vi "Hikvision 4004Hc EyeTraker.vi"() -> ()   [LabVIEW 2011]
uses:
  <vilib>/picture/picture.llb/imagedata.ctl
  <vilib>/Platform/TimedLoop/XDataNode/timing_clust.ctl
  <vilib>/Platform/TimedLoop/XDataNode/nitl_modes.ctl
  <vilib>/Platform/TimedLoop/XDataNode/wakeup.ctl
  <vilib>/Utility/file.llb/Read From Spreadsheet File (DBL).vi
  <vilib>/Utility/config.llb/Read Key (I32).vi
  <vilib>/Utility/config.llb/Read Key (U32).vi
  <vilib>/Utility/file.llb/Write To Spreadsheet File (DBL).vi
  <vilib>/Utility/config.llb/Write Key (I32).vi
  <vilib>/Utility/config.llb/Write Key (U32).vi
  <vilib>/Platform/TimedLoop/XDataNode/XDataNode.xnode
  <vilib>/Platform/TimedLoop/XDataNode/XDNodeRunTimeDep.lvlib
  <vilib>/Utility/config.llb/NI_LVConfig.lvlib
  <vilib>/vision/NI_Vision_Development_Module.lvlib
panel:
  out "XY图":cluster{dbl[], dbl[]}(graph)
  out "Histogram Graph":T1(graph) caption="直方图"
  in  "AviFileName":string="test9dots.avi"
  in  "method":enum16{"pupil", "CR", "pupil-CR"}(ring)=enum."pupil-CR"
  in  "bin":i32=10
  out "Frame Number":u32
  out "rectangle1":T2
  out "rectangle2":T2
  out "Image 2":T3(plugin-control)
  out "Image":T3(plugin-control)
  in  "VideoPara":cluster{"Brightness":i32, "Contrast":i32}={"Brightness"=128, "Contrast"=64} {"Contrast" min=0 max=127 scale=0.0..127.0; "Brightness" min=0 max=255 scale=0.0..255.0}
  out "valid fit 2":cluster{"CR Fit":bool, "pupil Fit":bool}
  out "valid fit":cluster{"CR Fit":bool, "pupil Fit":bool}
  in  "gaze Threshold1":dbl=2.0
  out "RAW循环持续时间":u64
  in  "blank of eye":T4={"NO. of Eyes"=0, "单选按钮"=enum."单选选项1", "eye1"=16711680, "eye2"=6618880} {"NO. of Eyes" items=["OneEye", "TwoEyes"]}
  out "数据处理循环持续时间 2":u64
  in  "CR Threshold 2":u8=240
  in  "Pupil Threshold 2":u8=75
  out "eye2":picture caption="新图片"
  in  "gaze Threshold 2":dbl=2.0
  out "gazing 2":bool
  in  "ImgResourse":u16(ring) items=["realeye", "avi"]
  out "gazing1":bool
  in  "Pupil Threshold1":u8=75
  in  "CR Threshold1":u8=240
  out "数据处理循环持续时间1":u64
  out "eye1":picture caption="新图片"
  out "new picture":picture caption="新图片"
  out "ROI循环持续时间":u64
  in  "停止":bool
  out "返回类型":i32
  out "ChannelOpen":u32 format="%x"
  out "GetTotalChannels":i32
  out "InitDSPs":i32
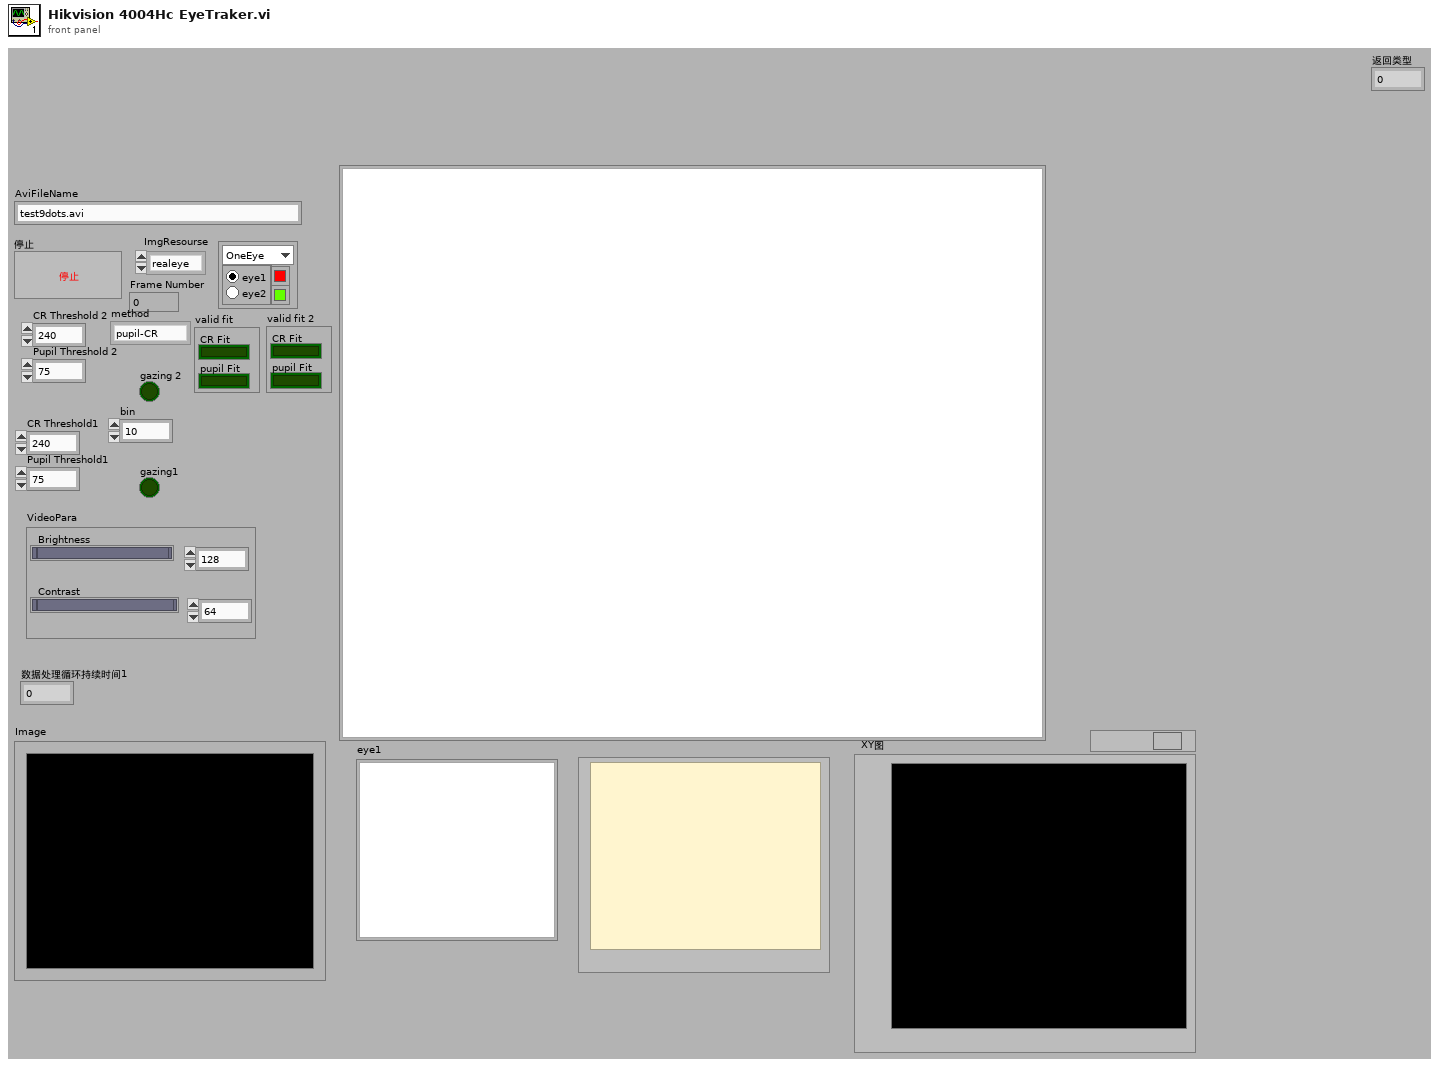
[diagram p1: front panel]
types:
  T1 = cluster{"X Values":dbl[], "Histogram: h(x)":i32[]}
  T2 = cluster{"value":i32, "value":i32, "value":i32, "value":i32}
  T3 = typedef "IMAQ Image.ctl" = refnum<image>
  T4 = cluster{"NO. of Eyes":u16, "单选按钮":enum32{"单选选项1", "单选选项2"}, "eye1":u32, "eye2":u32}
  T5 = typedef "XDNodeRunTimeDep.lvlib/timing_clust.ctl" = cluster{"Expected End [f-1]":u64, "Actual End [f-1]":u64, "Finished Late? [f-1]":bool, "Expected End [i-1]":u64, "Actual End [i-1]":u64, "Finished Late? [i-1]":bool, "Expected Start [i]":u64, "Actual Start [i]":u64, "Expected Start [f]":u64, "Actual Start [f]":u64, "Source Name":string, "Structure Name":string, "Period":i64, "Deadline":i64, "Offset":i64, "Start":i64, "Priority":i32, "Timeout":i32, "Mode":T6, "Wakeup Reason":T7, "Error":errorcluster, "Source Type":string, "Secondary Source Type":string, "Global End Time":u64, "Global Start Time":u64, "Frame Duration":u64, "Iteration Duration":u64, "Assigned CPU":i32, "I/O Scan Engine Mode":u32}
  T6 = typedef "XDNodeRunTimeDep.lvlib/nitl_modes.ctl" = enum32{"No Change", "Process missed periods, maintain original phase", "Discard missed periods, maintain original phase", "Process missed periods, ignore original phase", "Discard missed periods, ignore original phase"}
  T7 = typedef "XDNodeRunTimeDep.lvlib/wakeup.ctl" = enum32{"Normal", "Aborted", "Asynchronous wakeup", "Timing source error", "Timed loop error", "Timeout"}
  T8 = cluster{"pupil-CR array output":cluster{dbl[], dbl[]}, "CR array output":cluster{dbl[], dbl[]}, "pupil array output 3":cluster{dbl[], dbl[]}}
  T9 = typedef "NI_LVConfig.lvlib/Config Data RefNum.ctl" = refnum<k1>
  T10 = cluster{"ScreenWidth":i32, "ScreenHeight":i32, "distance":i32, "CameraDistance":i32, "AngleX":i32, "AngleY":i32}
  T11 = cluster{"CR":dbl[][], "pupil":dbl[][], "pupil-CR":dbl[][]}
  T12 = cluster{"CR":cluster{"平移参数":cluster{dbl, dbl}, "旋转参数":dbl, "y轴调整":dbl, "x曲面调整":dbl, "y曲面调整":dbl}, "pupil":cluster{"平移参数":cluster{dbl, dbl}, "旋转参数":dbl, "y轴调整":dbl, "x曲面调整":dbl, "y曲面调整":dbl}, "pupil-CR":cluster{"平移参数":cluster{dbl, dbl}, "旋转参数":dbl, "y轴调整":dbl, "x曲面调整":dbl, "y曲面调整":dbl}}
  T13 = typedef "Image Type" = u32
  T14 = typedef "imagedata.ctl" = cluster{"image type":i32, "image depth":i32, "image":u8[], "mask":u8[], "colors":u32[], "Rectangle":cluster{"left":i16, "top":i16, "right":i16, "bottom":i16}}
  T15 = cluster{"image subset":T14, "image subset":T14, bool}
  T16 = cluster{"CR Valid Fit":bool, "pupil Valid Fit":bool}
  T17 = cluster{"Minor Axis":cluster{"Point 1":cluster{"X":sgl, "Y":sgl}, "Point 2":cluster{"X":sgl, "Y":sgl}}, "Major Axis":cluster{"Point 1":cluster{"X":sgl, "Y":sgl}, "Point 2":cluster{"X":sgl, "Y":sgl}}, "输出簇":cluster{"point":cluster{"X":i32, "Y":i32}[], "Center":cluster{"X":sgl, "Y":sgl}}}
  T18 = cluster{"Point 1":cluster{"X":sgl, "Y":sgl}, "Point 2":cluster{"X":sgl, "Y":sgl}}
  T19 = typedef "AviRefnum.ctl" = refnum<k1>
  T20 = typedef "eventvkey.ctl" = enum16{"ASCII", "Enter", "Return", "Shift", "Ctrl", "Alt", "Cmd", "Opt", "Caps", "NumLock", "Clear", "Break", "Up", "Down", "Left", "Right", "Insert", "Delete", "Home", "End", "PageUp", "PageDown", "Escape", "Help", "Pause", "ScrollLock", "F1", "F2", "F3", "F4", "F5", "F6", "F7", "F8", "F9", "F10", "F11", "F12", "F13", "F14", "F15", "F16", "F17", "F18", "F19", "F20", "F21", "F22", "F23", "F24", "Play", "VolumeUp", "VolumeDown", "Mute", "Two Byte Char"}
  T21 = typedef "LVMouseTypeDef.ctl" = cluster{"Mouse Position":cluster{"X":i32, "Y":i32}, "Mouse Modifiers":cluster{"Button Down":bool, "Shift Mod":bool, "Menu Mod":bool, "Option Mod":bool}}
  T22 = cluster{"image subset":T14, "image subset":T14, "停止":bool}
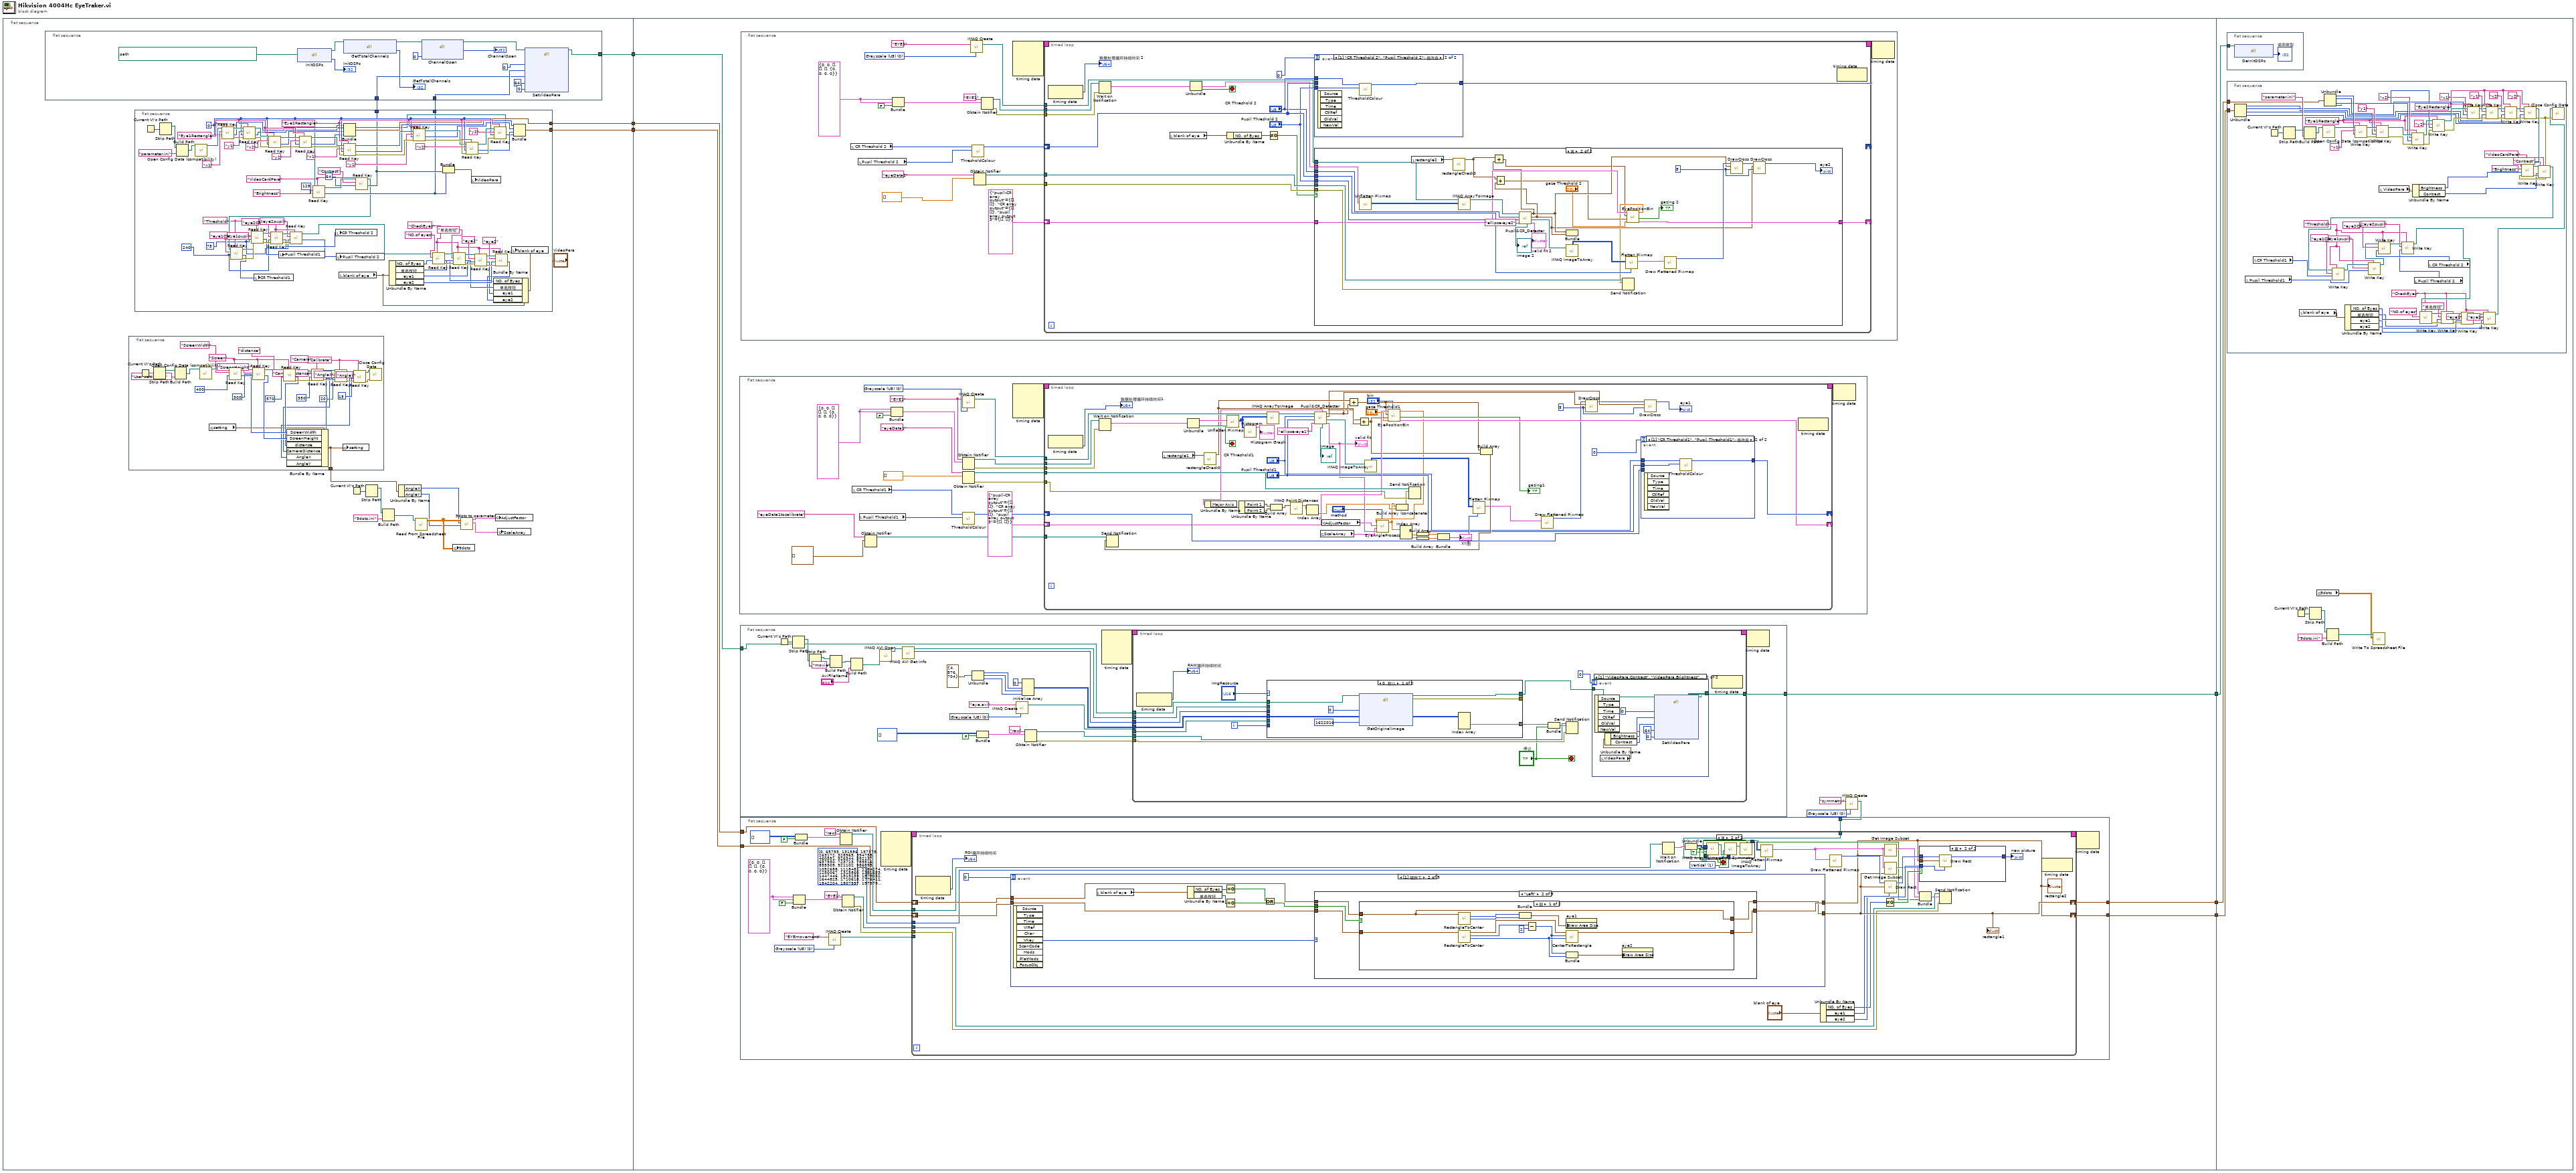
[diagram p0: block diagram]
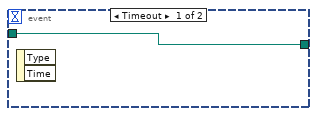
[diagram p2: hidden frame]
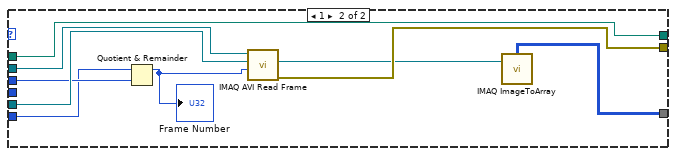
[diagram p3: hidden frame]
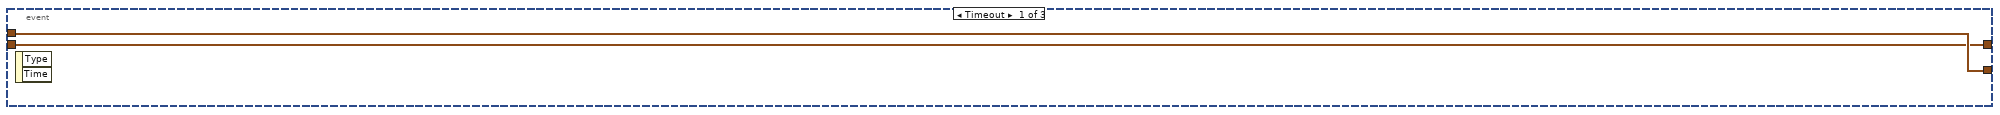
[diagram p6: hidden frame]
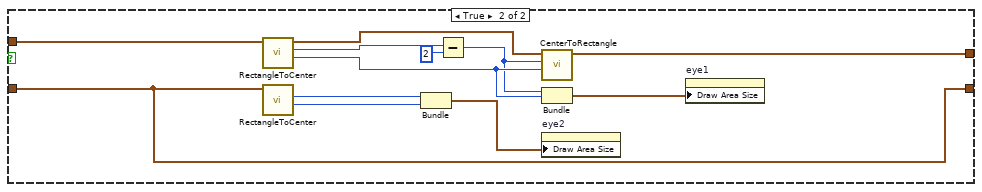
[diagram p8: hidden frame]
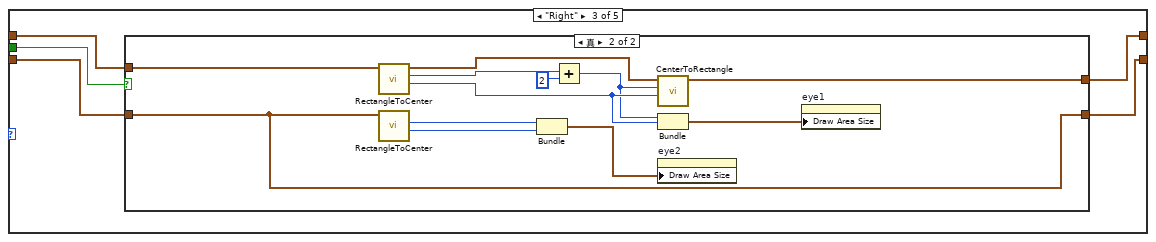
[diagram p9: hidden frame]
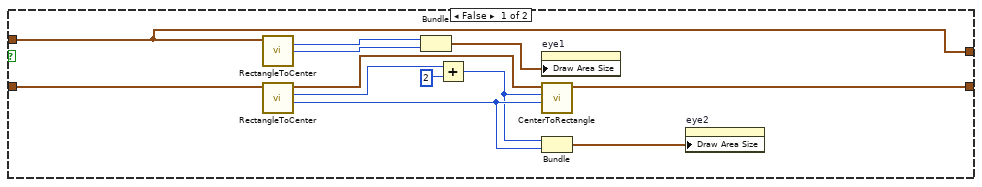
[diagram p10: hidden frame]
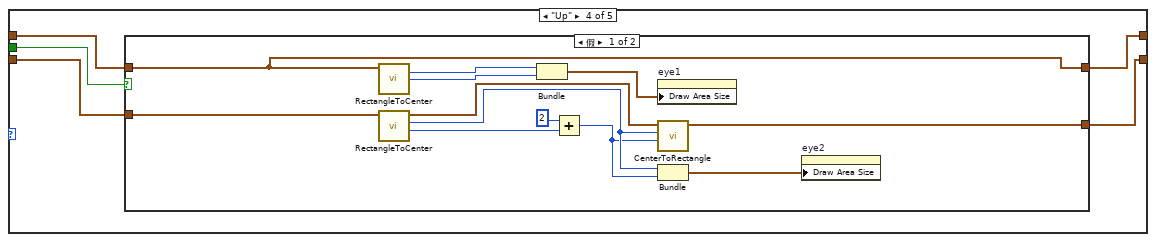
[diagram p11: hidden frame]
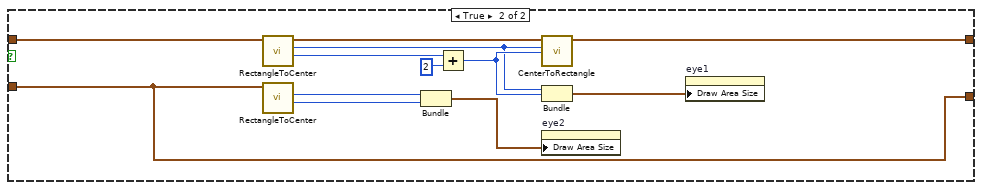
[diagram p12: hidden frame]
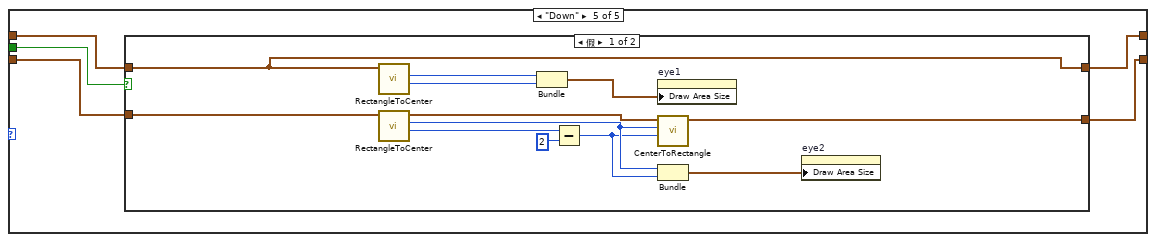
[diagram p13: hidden frame]
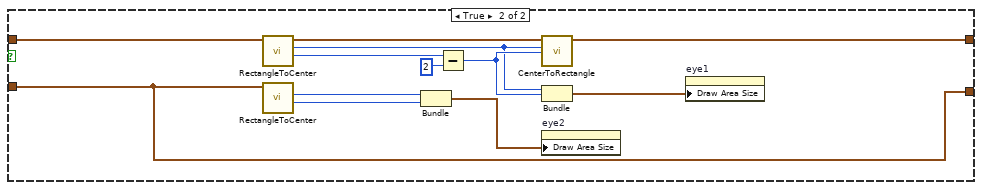
[diagram p14: hidden frame]
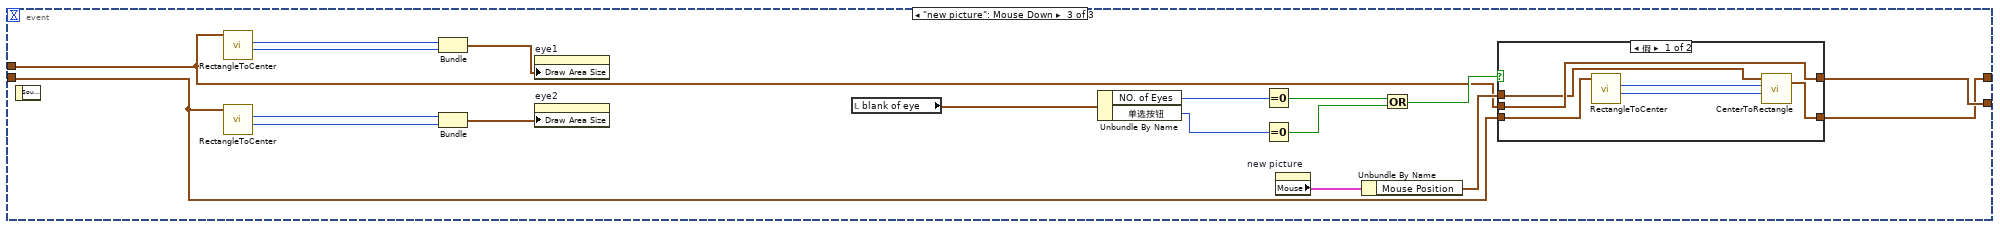
[diagram p15: hidden frame]
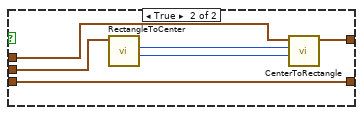
[diagram p16: hidden frame]
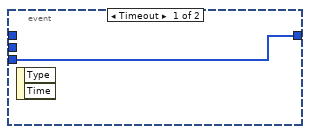
[diagram p17: hidden frame]
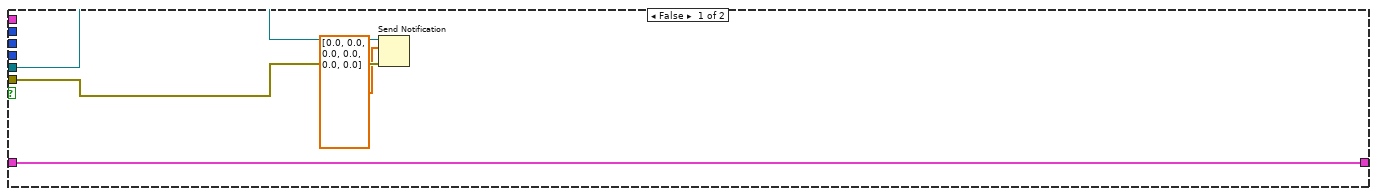
[diagram p18: hidden frame]
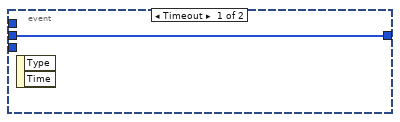
[diagram p19: hidden frame]
diagram:
  n1 = flat-sequence {
    tunnel: [w21] -> w6
    tunnel: [w20] -> w3
    tunnel: [w19] -> w2
    tunnel: w6 -> [w168]
    tunnel: [w172] -> w5
    tunnel: [w171] -> w4
    tunnel: w3 -> [w170]
    tunnel: w2 -> [w169]
    tunnel: [w167] -> w1
    tunnel: w5 -> [w654]
    tunnel: w4 -> [w653]
    tunnel: w1 -> [w652]
    frame #0 {
      n2 = flat-sequence {
        tunnel: [w66] -> w21
        tunnel: w18 -> [w60]
        tunnel: w17 -> [w61]
        frame #0 {
          n3 = dll-call lib="PTH1]abs CDocuments and Settingspan桌面workeye tracker\nHikvision Dll\nDs40xxSDK.dll" fn="InitDSPs"(path in=path "C:/Program Files/Hikvision/DS-4000系列板卡SDK and Demo Version 5.1/SDK/card sdk/Ds40xxSDK.dll" ("dll路径输入")) -> (path out=w68:path, "返回类型"=→"InitDSPs":i32)  [unwired: 2 in, 1 out]
          n4 = dll-call lib="PTH1]abs CDocuments and Settingspan桌面workeye tracker\nHikvision Dll\nDs40xxSDK.dll" fn="GetTotalChannels"(path in=w68) -> (path out=w70:path, "返回类型"=→"GetTotalChannels":i32)  [unwired: 2 in, 1 out]
          n5 = dll-call lib="PTH1]abs CDocuments and Settingspan桌面workeye tracker\nHikvision Dll\nDs40xxSDK.dll" fn="ChannelOpen"(path in=w70, "ChannelNum"=0) -> (path out=w65:path, "返回类型"=→"ChannelOpen":u32)  [unwired: 3 in, 1 out]
          n6 = dll-call lib="PTH1babs C\nProgram Files\tHikvision+DS-4000系列板卡SDK and Demo Version 5.1Bin\nDs40xxSDK.dll" fn="SetVideoPara"(path in=w65, "hChannelHandle"=u32 0, "Brightness"=w61, "Contrast"=w60, "Saturation"=64, "Hue"=0) -> (path out=w66:path)  [unwired: 7 in, 2 out]
        }
      }
      n7 = flat-sequence {
        tunnel: [w23] -> w9
        frame #0 {
          w30 = "Calibrate" ("section")
          w49 = "Screen" ("section")
          n8 = Current VI's Path() -> (path=w58:path)
          n9 = Strip Path(path=w58) -> (stripped path=w59:path)  [unwired: 1 out]
          n10 = Build Path(base path=w59, name or relative path="User Setting.ini" ("名称或相对路径")) -> (appended path=w56:path)
          n11 = call <vilib>:"Open Config Data (compatibility).vi"("configuration file path"=w56) -> ("refnum"=w55:T9)  [unwired: 8 in, 2 out]
          n12 = global read "全局 1.vi" "setting"() -> (w22:T10)
          n13 = call-poly <vilib>:"Read Key.vi"("section"=w49, "default value"=400 ("Pupil Threshold1"), "key"="ScreenWidth", "refnum"=w55) -> ("value"=w40:i32, "refnum out"=w53:T9)  [unwired: 1 in, 5 out]
          n14 = call-poly <vilib>:"Read Key.vi"("section"=w49, "default value"=300 ("Pupil Threshold1"), "key"="ScreenHeight", "refnum"=w53) -> ("value"=w39:i32, "refnum out"=w52:T9)  [unwired: 1 in, 5 out]
          n15 = call-poly <vilib>:"Read Key.vi"("section"=w49, "default value"=570 ("Pupil Threshold1"), "key"="distance", "refnum"=w52) -> ("error out"=w47:errorcluster, "value"=w38:i32, "refnum out"=w48:T9)  [unwired: 1 in, 4 out]
          n16 = call-poly <vilib>:"Read Key.vi"("section"="Camera", "error in (no error)"=w47, "default value"=350 ("Pupil Threshold1"), "key"="CameraDistance", "refnum"=w48) -> ("error out"=w37:errorcluster, "value"=w36:i32, "refnum out"=w35:T9)  [unwired: 4 out]
          n17 = call-poly <vilib>:"Read Key.vi"("section"=w30, "error in (no error)"=w37, "default value"=20 ("Pupil Threshold1"), "key"="AngleX", "refnum"=w35) -> ("error out"=w33:errorcluster, "value"=w25:i32, "refnum out"=w34:T9)  [unwired: 4 out]
          n18 = call-poly <vilib>:"Read Key.vi"("section"=w30, "error in (no error)"=w33, "default value"=15 ("Pupil Threshold1"), "key"="AngleY", "refnum"=w34) -> ("error out"=w31:errorcluster, "value"=w24:i32, "refnum out"=w32:T9)  [unwired: 4 out]
          n19 = Bundle By Name(cluster=w22, "ScreenWidth"=w40, "ScreenHeight"=w39, "distance"=w38, "CameraDistance"=w36, "AngleX"=w25, "AngleY"=w24) -> (w23:T10)
          n20 = global write "全局 1.vi" "setting"(w23) -> ()
          n21 = call <vilib>:"Close Config Data.vi"("error in (no error)"=w31, "refnum"=w32) -> ()  [unwired: 1 in, 9 out]
        }
      }
      n22 = flat-sequence {
        tunnel: [w125] -> w20
        tunnel: [w124] -> w19
        tunnel: [w116] -> w18
        tunnel: [w115] -> w17
        frame #0 {
          w74 = "CheckEyes" ("section")
          w98 = 75
          w100 = 240
          w106 = "Threshold" ("section")
          w121 = "VideoCardPara" ("section")
          w134 = 0
          w153 = "Eye2Rectangle" ("section")
          w148 = "Eye1Rectangle" ("section")
          n23 = Current VI's Path() -> (path=w135:path)
          n24 = Strip Path(path=w135) -> (stripped path=w136:path)  [unwired: 1 out]
          n25 = Build Path(base path=w136, name or relative path="parameter.ini" ("名称或相对路径")) -> (appended path=w138:path)
          n26 = call <vilib>:"Open Config Data (compatibility).vi"("configuration file path"=w138) -> ("refnum"=w139:T9)  [unwired: 8 in, 2 out]
          n27 = call-poly <vilib>:"Read Key.vi"("section"=w148, "default value"=w134, "key"="x1", "refnum"=w139) -> ("error out"=w141:errorcluster, "value"=w133:i32, "refnum out"=w142:T9)  [unwired: 1 in, 4 out]
          n28 = call-poly <vilib>:"Read Key.vi"("section"=w148, "error in (no error)"=w141, "default value"=w134, "key"="y1", "refnum"=w142) -> ("error out"=w144:errorcluster, "value"=w132:i32, "refnum out"=w145:T9)  [unwired: 4 out]
          n29 = call-poly <vilib>:"Read Key.vi"("section"=w148, "error in (no error)"=w144, "default value"=w134, "key"="x2", "refnum"=w145) -> ("error out"=w146:errorcluster, "value"=w131:i32, "refnum out"=w147:T9)  [unwired: 4 out]
          n30 = call-poly <vilib>:"Read Key.vi"("section"=w148, "error in (no error)"=w146, "default value"=w134, "key"="y2", "refnum"=w147) -> ("error out"=w163:errorcluster, "value"=w130:i32, "refnum out"=w162:T9)  [unwired: 4 out]
          n31 = local read "blank of eye"() -> (w81:T4)
          n32 = Bundle("value"=w133, "value"=w132, "value"=w131, "value"=w130) -> (w125:T2)  [unwired: 1 out]
          n33 = call-poly <vilib>:"Read Key.vi"("section"=w153, "error in (no error)"=w163, "default value"=w134, "key"="x1", "refnum"=w162) -> ("error out"=w160:errorcluster, "value"=w129:i32, "refnum out"=w159:T9)  [unwired: 4 out]
          n34 = Unbundle By Name(w81) -> ("NO. of Eyes"=w85:u16, "单选按钮"=w84:enum32{"单选选项1", "单选选项2"}, "eye1"=w83:u32, "eye2"=w82:u32)
          n35 = call-poly <vilib>:"Read Key.vi"("section"=w153, "error in (no error)"=w160, "default value"=w134, "key"="y1", "refnum"=w159) -> ("error out"=w157:errorcluster, "value"=w128:i32, "refnum out"=w156:T9)  [unwired: 4 out]
          n36 = call-poly <vilib>:"Read Key.vi"("section"=w153, "error in (no error)"=w157, "default value"=w134, "key"="x2", "refnum"=w156) -> ("error out"=w155:errorcluster, "value"=w127:i32, "refnum out"=w154:T9)  [unwired: 4 out]
          n37 = call-poly <vilib>:"Read Key.vi"("section"=w153, "error in (no error)"=w155, "default value"=w134, "key"="y2", "refnum"=w154) -> ("value"=w126:i32, "refnum out"=w123:T9)  [unwired: 5 out]
          n38 = call-poly <vilib>:"Read Key.vi"("section"=w121, "default value"=128, "key"="Brightness", "refnum"=w123) -> ("value"=w115:i32, "refnum out"=w120:T9)  [unwired: 1 in, 5 out]
          n39 = call-poly <vilib>:"Read Key.vi"("section"=w121, "default value"=64, "key"="Contrast", "refnum"=w120) -> ("value"=w116:i32, "refnum out"=w107:T9)  [unwired: 1 in, 5 out]
          n40 = call-poly <vilib>:"Read Key.vi"("section"=w106, "default value"=w100, "key"="eye1CR", "refnum"=w107) -> ("error out"=w113:errorcluster, "value"=w103:i32, "refnum out"=w112:T9)  [unwired: 1 in, 4 out]
          n41 = call-poly <vilib>:"Read Key.vi"("section"=w106, "error in (no error)"=w113, "default value"=w98, "key"="eye1pupil", "refnum"=w112) -> ("error out"=w111:errorcluster, "value"=w102:i32, "refnum out"=w110:T9)  [unwired: 4 out]
          n42 = local write "CR Threshold1"(w103) -> ()
          n43 = call-poly <vilib>:"Read Key.vi"("section"=w106, "error in (no error)"=w111, "default value"=w100, "key"="eye2CR", "refnum"=w110) -> ("error out"=w109:errorcluster, "value"=w99:i32, "refnum out"=w108:T9)  [unwired: 4 out]
          n44 = local write "Pupil Threshold1"(w102) -> ()
          n45 = call-poly <vilib>:"Read Key.vi"("section"=w106, "error in (no error)"=w109, "default value"=w98, "key"="eye2pupil", "refnum"=w108) -> ("value"=w96:i32, "refnum out"=w75:T9)  [unwired: 5 out]
          n46 = local write "CR Threshold 2"(w99) -> ()
          n47 = local write "Pupil Threshold 2"(w96) -> ()
          n48 = call-poly <vilib>:"Read Key.vi"("section"=w74, "default value"=w85, "key"="NO.of eyes", "refnum"=w75) -> ("error out"=w89:errorcluster, "value"=w79:u32, "refnum out"=w90:T9)  [unwired: 1 in, 4 out]
          n49 = Bundle("value"=w115, "value"=w116) -> (w114:cluster{"value":i32, "value":i32})  [unwired: 1 out]
          n50 = call-poly <vilib>:"Read Key.vi"("section"=w74, "error in (no error)"=w89, "default value"=w84, "key"="单选按钮", "refnum"=w90) -> ("error out"=w94:errorcluster, "value"=w78:i32, "refnum out"=w93:T9)  [unwired: 4 out]
          n51 = local write "VideoPara"(w114) -> ()
          n52 = call-poly <vilib>:"Read Key.vi"("section"=w74, "error in (no error)"=w94, "default value"=w83, "key"="eye1", "refnum"=w93) -> ("error out"=w92:errorcluster, "value"=w77:u32, "refnum out"=w91:T9)  [unwired: 4 out]
          n53 = call-poly <vilib>:"Read Key.vi"("section"=w74, "error in (no error)"=w92, "default value"=w82, "key"="eye2", "refnum"=w91) -> ("value"=w76:u32)  [unwired: 6 out]
          n54 = Bundle By Name(cluster=w81, "NO. of Eyes"=w79, "单选按钮"=w78, "eye1"=w77, "eye2"=w76) -> (w80:T4)
          n55 = local write "blank of eye"(w80) -> ()
          n56 = Bundle("value"=w129, "value"=w128, "value"=w127, "value"=w126) -> (w124:T2)  [unwired: 1 out]
        }
      }
      n57 = Current VI's Path() -> (path=w12:path)
      n58 = Strip Path(path=w12) -> (stripped path=w13:path)  [unwired: 1 out]
      n59 = Build Path(base path=w13, name or relative path="9dots.ini" ("名称或相对路径")) -> (appended path=w10:path)
      n60 = Unbundle By Name(w9) -> ("AngleX"=w8:i32, "AngleY"=w7:i32)
      n61 = call-poly <vilib>:"Read From Spreadsheet File.vi"("file path (dialog if empty)"=w10) -> ("all rows"=w11:dbl[][])  [unwired: 3 in, 7 out]
      n62 = global write "全局 1.vi" "9dots"(w11) -> ()
      n63 = call "9dots to parameter.vi"("yDegree"=w7, "xDegree"=w8, "9dots"=w11) -> ("ScaleArray"=w15:T11, "adjutFactor"=w16:T12)  [unwired: 7 out]
      n64 = global write "全局 1.vi" "AdjustFactor"(w16) -> ()
      n65 = global write "全局 1.vi" "ScaleArray"(w15) -> ()
    }
    frame #1 {
      w164 = T13 0 items=["Grayscale (U8)", "Grayscale (I16)", "Grayscale (SGL)", "Complex (CSG)", "RGB (U32)", "HSL (U32)", "RGB (U64)", "Grayscale (U16)"] ("Image Type")
      n66 = flat-sequence {
        frame #0 {
          w493 = T13 0 items=["Grayscale (U8)", "Grayscale (I16)", "Grayscale (SGL)", "Complex (CSG)", "RGB (U32)", "HSL (U32)", "RGB (U64)", "Grayscale (U16)"] ("Image Type")
          w489 = "EYE1" ("Image Name")
          w488 = T14 {"image type"=0, "image depth"=0, "image"=[], "mask"=[], "colors"=[], "Rectangle"={"left"=0, "top"=0, "right"=0, "bottom"=0}} ("image subset")
          n67 = local read "CR Threshold1"() -> (w494:u8)
          n68 = local read "Pupil Threshold1"() -> (w495:u8)
          n69 = Obtain Notifier(name (unnamed)="eyeData1tocalibrate" ("Image Name"), notification data type=cluster{sgl, sgl}[] [] ("添加的数组")) -> (notifier out=w480:refnum<notifier>)  [unwired: 2 in, 2 out]
          n70 = Bundle("image subset"=w488, "image subset"=w488, FALSE) -> (w491:T15)  [unwired: 1 out]
          n71 = call "IMAQ Create"("Image Name"=w489, "Image Type"=w493) -> ("New Image"=w492:T3)  [unwired: 2 in, 2 out]
          n72 = Obtain Notifier(name (unnamed)=w489, notification data type=w491) -> (notifier out=w484:refnum<notifier>, error out=w483:errorcluster)  [unwired: 2 in, 1 out]
          n73 = Obtain Notifier(name (unnamed)="eyeData1" ("Image Name"), notification data type=dbl[] [] ("添加的数组")) -> (notifier out=w486:refnum<notifier>, error out=w485:errorcluster)  [unwired: 2 in, 1 out]
          n74 = call "ThresholdColour.vi"("Pupil Threshold"=w495, "HighLight Spot Threshold"=w494) -> ("colors"=w490:u32[])  [unwired: 9 out]
          n75 = node-c288() -> (w498:T5)  [unwired: 4 out]
          n76 = timed-loop {
            timing: w498 -> [_]
            timing-out: [_] -> w497
            tunnel: w484 -> [w556]
            tunnel: w483 -> [w555]
            shift-right: [w554] -> _
            shift-left: w490 -> [w553]
            tunnel: w492 -> [w552]
            tunnel: w486 -> [w550]
            tunnel: w485 -> [w549]
            shift-right: [w547] -> _
            shift-left: T8 {"pupil-CR array output"={[], []}, "CR array output"={[], []}, "pupil array output 3"={[], []}} ("data array output") -> [w548]
            tunnel: w480 -> [w546]
            stop <- w551 stop-if-true
            w509 = 5 ("pixel")
            n77 = node-c288() -> (→"数据处理循环持续时间1":i64)  [unwired: 1 out]
            n78 = Wait on Notification(notifier=w556, error in (no error)=w555) -> (notification=w544:T15)  [unwired: 5 out]
            n79 = local read "rectangle1"() -> (w532:T2)
            n80 = Unbundle(w544) -> ("image subset"=w541:T14, w551:bool)  [unwired: 1 out]
            n81 = call "rectangleCheck0.vi"("rectangle"=w532) -> ("rectangle out"=w531:cluster{"x1":i32, "y1":i32})  [unwired: 10 out]
            n82 = call <vilib>:"Unflatten Pixmap.vi"("image data"=w541) -> ("8-bit pixmap"=w514:u8[][])  [unwired: 10 out]
            n83 = call "Histogram.vi"("8-bit pixmap"=w514) -> ("Histogram Graph"=→"Histogram Graph":T1)  [unwired: 10 out]
            n84 = call "IMAQ ArrayToImage"("Image Pixels (U8)"=w514, "Image"=w552) -> ("Image Out"=w540:T3)  [unwired: 4 in, 5 out]
            n85 = call "Pupil&CR_Detecter.vi"("Image Name"="ellipse-eye1", "Pupil Threshold"="Pupil Threshold1", "HighLight Spot Threshold"="CR Threshold1", "image input"=w540) -> ("valid fit"=w526:T16, "Image Dst Out"=w537:T3, "pupil Circles Data"=w529:cluster{"Pos. X":sgl, "Pos. Y":sgl}, "CR Circles Data"=w530:cluster{"Pos. X":sgl, "Pos. Y":sgl}, "Image Out"=→"Image":T3, "Axis"=w507:T17)  [unwired: 2 out]
            "valid fit" <- w526
            n86 = Unbundle By Name(w507) -> ("Major Axis"=w506:T18)
            n87 = Unbundle By Name(w506) -> ("Point 1"=w505:cluster{"X":sgl, "Y":sgl}, "Point 2"=w504:cluster{"X":sgl, "Y":sgl})
            n88 = Build Array(w505, w504) -> (w503:cluster{"X":sgl, "Y":sgl}[])
            n89 = call "IMAQ Point Distances"("Points"=w503) -> ("Distances"=w502:sgl[])  [unwired: 1 in, 4 out]
            n90 = Index Array(array=w502) -> (element=w500:sgl)  [unwired: 1 in]
            n91 = global read "全局 1.vi" "ScaleArray"() -> (w523:T11)
            n92 = global read "全局 1.vi" "AdjustFactor"() -> (w524:T12)
            n93 = Add(x=w531, y=w530) -> (x+y=w528:cluster{sgl, sgl})
            n94 = Add(x=w529, y=w531) -> (x+y=w527:cluster{sgl, sgl})
            n95 = call "IMAQ ImageToArray"("Image"=w537) -> ("Image Pixels (U8)"=w536:u8[][])  [unwired: 2 in, 5 out]
            n96 = call "EyePositionBin.vi"("bin"="bin", "gaze Threshold"="gaze Threshold1", "pupil input"=w527, "CR input"=w528, "data array input"=w548) -> ("data array output"=w547:T8, "gaze"=→"gazing1":bool, "eyeposition array"=w525:dbl[])  [unwired: 4 out]
            n97 = call "EyeAngleProcess.vi"("method"="method", "valid fit"=w526, "ScaleArray"=w523, "AdjustFactor"=w524, "EYEDateArray"=w525) -> ("EyeAngle"=w501:dbl[])  [unwired: 6 out]
            n98 = Build Array (concatenate)(w501, w500) -> (w499:dbl[])
            n99 = Index Array(array=w501) -> (element #1=w521:dbl, element #2=w520:dbl)  [unwired: 2 in]
            n100 = Send Notification(notification=w499, notifier=w550, error in (no error)=w549) -> ()  [unwired: 2 out]
            n101 = Build Array(w521) -> (w519:dbl[])
            n102 = Build Array(w520) -> (w518:dbl[])
            n103 = Bundle(w519, w518) -> (→"XY图":cluster{dbl[], dbl[]})  [unwired: 1 out]
            n104 = call <vilib>:"Flatten Pixmap.vi"("colors"=w553, "8-bit pixmap"=w536) -> ("image data"=w542:T14)  [unwired: 4 in, 5 out]
            n105 = Build Array(w528, w527) -> (w543:cluster{sgl, sgl}[])
            n106 = Send Notification(notification=w543, notifier=w546) -> ()  [unwired: 1 in, 2 out]
            n107 = call <vilib>:"Draw Flattened Pixmap.vi"("image data"=w542) -> ("new picture"=w515:picture)  [unwired: 1 in, 7 out]
            n108 = call "DrawCross.vi"("pixel"=w509, "position"=w530, "picture input"=w515) -> ("picture Output"=w510:picture)  [unwired: 1 in, 7 out]
            n109 = event shown="[1] \"CR Threshold1\", \"Pupil Threshold1\": 值改变" {
              selector: _ -> [_ _]
              dyn-events: _ -> [_ _]
              timeout: 0 -> [_ _]
              tunnel: "CR Threshold1" -> [_ w560]
              tunnel: "Pupil Threshold1" -> [_ w559]
              tunnel: [w557 w558] -> w554
              tunnel: w553 -> [w557 _]
              event Timeout {
                n110 = event-data() -> ()  [unwired: 3 out]
              }
              event "CR Threshold1", "Pupil Threshold1": Value Change {
                n111 = event-data() -> ()  [unwired: 7 out]
                n112 = call "ThresholdColour.vi"("Pupil Threshold"=w559, "HighLight Spot Threshold"=w560) -> ("colors"=w558:u32[])  [unwired: 9 out]
              }
            }
            n113 = call "DrawCross.vi"("pixel"=w509, "position"=w529, "picture input"=w510) -> ("picture Output"=→"eye1":picture)  [unwired: 1 in, 7 out]
            n114 = node-c288() -> ()  [unwired: 2 out]
          }
          n115 = node-c288(w497) -> ()  [unwired: 1 out]
        }
      }
      n116 = flat-sequence {
        tunnel: w168 -> [w190]
        tunnel: [w185] -> w167
        frame #0 {
          w194 = T13 0 items=["Grayscale (U8)", "Grayscale (I16)", "Grayscale (SGL)", "Complex (CSG)", "RGB (U32)", "HSL (U32)", "RGB (U64)", "Grayscale (U16)"] ("Image Type")
          n117 = Current VI's Path() -> (path=w180:path)
          n118 = Strip Path(path=w180) -> (stripped path=w179:path)  [unwired: 1 out]
          n119 = Strip Path(path=w179) -> (stripped path=w178:path)  [unwired: 1 out]
          n120 = Build Path(base path=w178, name or relative path="movie" ("名称或相对路径")) -> (appended path=w175:path)
          n121 = Build Path(base path=w175, name or relative path="AviFileName") -> (appended path=w174:path)
          n122 = call "IMAQ AVI Open"("AVI Path"=w174) -> ("Avi Refnum"=w173:T19)  [unwired: 1 in, 9 out]
          n123 = call "IMAQ AVI Get Info"("Avi Refnum"=w173) -> ("Number of Frames"=w192:u32, "Avi Refnum (duplicate)"=w191:T19)  [unwired: 1 in, 8 out]
          n124 = Unbundle(cluster{"元素":i32, "元素 2":i32, "元素 3":i32} {"元素"=4, "元素 2"=576, "元素 3"=704}) -> ("元素"=w197:i32, "元素 2"=w196:i32, "元素 3"=w195:i32)
          n125 = Bundle("Image Pixels (U8)"=u8[][] [], "停止"=FALSE) -> (w182:cluster{"Image Pixels (U8)":u8[][], "停止":bool})  [unwired: 1 out]
          n126 = call "IMAQ Create"("Image Name"="eye.avi", "Image Type"=w194) -> ("New Image"=w188:T3)  [unwired: 2 in, 2 out]
          n127 = Initialize Array(u8 0 ("元素"), w197, w196, w195) -> (w189:u8[][][])
          n128 = Obtain Notifier(name (unnamed)="raw" ("Image Name"), notification data type=w182) -> (notifier out=w181:refnum<notifier>, error out=w186:errorcluster)  [unwired: 2 in, 1 out]
          n129 = node-c288() -> (w201:T5)  [unwired: 4 out]
          n130 = timed-loop {
            timing: w201 -> [_]
            timing-out: [_] -> w200
            tunnel: w192 -> [w215]
            tunnel: w191 -> [w214]
            tunnel: w190 -> [w213]
            tunnel: w189 -> [w212]
            tunnel: w188 -> [w211]
            tunnel: w181 -> [w210]
            tunnel: w186 -> [w209]
            tunnel: [w204] -> w185
            i -> [w216]
            stop <- "停止" stop-if-true
            n131 = node-c288() -> (→"RAW循环持续时间":i64)  [unwired: 1 out]
            n132 = case shown="0, 默认" "ImgResourse" {
              tunnel: w212 -> [w234 _]
              tunnel: [w232 w243] -> _
              tunnel: [w231 w237] -> w207
              tunnel: w214 -> [_ w242]
              tunnel: w211 -> [_ w241]
              tunnel: w215 -> [_ w240]
              tunnel: w216 -> [_ w239]
              tunnel: w213 -> [w230 w236]
              tunnel: [w229 w236] -> w203
              frame 0, Default {
                n133 = dll-call lib="PTH1]abs CDocuments and Settingspan桌面workeye tracker\nHikvision Dll\nDs40xxSDK.dll" fn="GetOriginalImage"(path in=w230, "hChannelHandle"=u32 0, "ImageBuf"=w234, "Size"=u32 1622016) -> (path out=w229:path, error out=w232:errorcluster, "ImageBuf"=w233:u8[][][])  [unwired: 3 in, 2 out]
                n134 = Index Array(array=w233) -> (element=w231:u8[][])  [unwired: 3 in]
              }
              frame 1 {
                n135 = Quotient & Remainder(x=w239, y=w240) -> (x-y*floor(x/y)=w235:u32)  [unwired: 1 out]
                "Frame Number" <- w235
                n136 = call "IMAQ AVI Read Frame"("Frame Number"=w235, "Image"=w241, "Avi Refnum"=w242) -> ("error out"=w243:errorcluster, "Image Out"=w238:T3)  [unwired: 2 in, 5 out]
                n137 = call "IMAQ ImageToArray"("Image"=w238) -> ("Image Pixels (U8)"=w237:u8[][])  [unwired: 2 in, 5 out]
              }
            }
            n138 = Bundle("Image Pixels (U8)"=w207, "停止"="停止") -> (w206:cluster{"Image Pixels (U8)":u8[][], "停止":bool})  [unwired: 1 out]
            n139 = Send Notification(notification=w206, notifier=w210, error in (no error)=w209) -> ()  [unwired: 2 out]
            n140 = event shown="[1] \"VideoPara.Contrast\", \"VideoPara.Brightness\": 值改变" {
              selector: _ -> [_ _]
              dyn-events: _ -> [_ _]
              timeout: 0 -> [_ _]
              tunnel: w203 -> [w218 w226]
              tunnel: [w218 w225] -> w204
              event Timeout {
                n141 = event-data() -> ()  [unwired: 3 out]
              }
              event "VideoPara.Contrast", "VideoPara.Brightness": Value Change {
                n142 = event-data() -> ()  [unwired: 7 out]
                n143 = local read "VideoPara"() -> (w221:cluster{"Brightness":i32, "Contrast":i32})
                n144 = Unbundle By Name(w221) -> ("Brightness"=w220:i32, "Contrast"=w219:i32)
                n145 = dll-call lib="PTH1babs C\nProgram Files\tHikvision+DS-4000系列板卡SDK and Demo Version 5.1Bin\nDs40xxSDK.dll" fn="SetVideoPara"(path in=w226, "hChannelHandle"=u32 0, "Brightness"=w220, "Contrast"=w219, "Saturation"=64, "Hue"=0) -> (path out=w225:path)  [unwired: 7 in, 2 out]
              }
            }
            n146 = node-c288() -> ()  [unwired: 2 out]
          }
          n147 = node-c288(w200) -> ()  [unwired: 1 out]
        }
      }
      n148 = flat-sequence {
        tunnel: [w264] -> w172
        tunnel: [w263] -> w171
        tunnel: w170 -> [w262]
        tunnel: w169 -> [w261]
        tunnel: w166 -> [w249]
        frame #0 {
          w257 = T14 {"image type"=0, "image depth"=0, "image"=[], "mask"=[], "colors"=[], "Rectangle"={"left"=0, "top"=0, "right"=0, "bottom"=0}} ("image subset")
          w267 = T13 0 items=["Grayscale (U8)", "Grayscale (I16)", "Grayscale (SGL)", "Complex (CSG)", "RGB (U32)", "HSL (U32)", "RGB (U64)", "Grayscale (U16)"] ("Image Type")
          n149 = Bundle("image subset"=w257, "image subset"=w257, FALSE) -> (w259:T15)  [unwired: 1 out]
          n150 = Bundle("Image Pixels (U8)"=u8[][] [], "停止"=FALSE) -> (w254:cluster{"Image Pixels (U8)":u8[][], "停止":bool})  [unwired: 1 out]
          n151 = call "IMAQ Create"("Image Name"="EYEmovement", "Image Type"=w267) -> ("New Image"=w265:T3)  [unwired: 2 in, 2 out]
          n152 = Obtain Notifier(name (unnamed)="raw" ("Image Name"), notification data type=w254) -> (notifier out=w250:refnum<notifier>)  [unwired: 2 in, 2 out]
          n153 = Obtain Notifier(name (unnamed)="EYE1" ("Image Name"), notification data type=w259) -> (notifier out=w256:refnum<notifier>, error out=w255:errorcluster)  [unwired: 2 in, 1 out]
          n154 = node-c288() -> (w270:T5)  [unwired: 4 out]
          n155 = timed-loop {
            timing: w270 -> [_]
            timing-out: [_] -> w269
            tunnel: u32[] [0, 65793, 131586, 197379, 263172, 328965, 394758, 460551, 526344, 592137, 657930, 723723, 789516, 855309, 921102, 986895, 1052688, 1118481, 1184274, 1250067, 1315860, 1381653, 1447446, 1513239, 1579032, 1644825, 1710618, 1776411, 1842204, 1907997, 1973790, 2039583, 2105376, 2171169, 2236962, 2302755, 2368548, 2434341, 2500134, 2565927, 2631720, 2697513, 2763306, 2829099, 2894892, 2960685, 3026478, 3092271, 3158064, 3223857, 3289650, 3355443, 3421236, 3487029, 3552822, 3618615, 3684408, 3750201, 3815994, 3881787, 3947580, 4013373, 4079166, 4144959, 4210752, 4276545, 4342338, 4408131, 4473924, 4539717, 4605510, 4671303, 4737096, 4802889, 4868682, 4934475, 5000268, 5066061, 5131854, 5197647, 5263440, 5329233, 5395026, 5460819, 5526612, 5592405, 5658198, 5723991, 5789784, 5855577, 5921370, 5987163, 6052956, 6118749, 6184542, 6250335, 6316128, 6381921, 6447714, 6513507, 6579300, 6645093, 6710886, 6776679, 6842472, 6908265, 6974058, 7039851, 7105644, 7171437, 7237230, 7303023, 7368816, 7434609, 7500402, 7566195, 7631988, 7697781, 7763574, 7829367, 7895160, 7960953, 8026746, 8092539, 8158332, 8224125, 8289918, 8355711, 8421504, 8487297, 8553090, 8618883, 8684676, 8750469, 8816262, 8882055, 8947848, 9013641, 9079434, 9145227, 9211020, 9276813, 9342606, 9408399, 9474192, 9539985, 9605778, 9671571, 9737364, 9803157, 9868950, 9934743, 10000536, 10066329, 10132122, 10197915, 10263708, 10329501, 10395294, 10461087, 10526880, 10592673, 10658466, 10724259, 10790052, 10855845, 10921638, 10987431, 11053224, 11119017, 11184810, 11250603, 11316396, 11382189, 11447982, 11513775, 11579568, 11645361, 11711154, 11776947, 11842740, 11908533, 11974326, 12040119, 12105912, 12171705, 12237498, 12303291, 12369084, 12434877, 12500670, 12566463, 12632256, 12698049, 12763842, 12829635, 12895428, 12961221, 13027014, 13092807, 13158600, 13224393, 13290186, 13355979, 13421772, 13487565, 13553358, 13619151, 13684944, 13750737, 13816530, 13882323, 13948116, 14013909, 14079702, 14145495, 14211288, 14277081, 14342874, 14408667, 14474460, 14540253, 14606046, 14671839, 14737632, 14803425, 14869218, 14935011, 15000804, 15066597, 15132390, 15198183, 15263976, 15329769, 15395562, 15461355, 15527148, 15592941, 15658734, 15724527, 15790320, 15856113, 15921906, 15987699, 16053492, 16119285, 16185078, 16250871, 16316664, 16382457, 16448250, 16514043, 16579836, 16645629, 16711422, 16777215] ("colors") -> [w298]
            shift-right: [w294] -> w264
            shift-left: w262 -> [w296]
            tunnel: w256 -> [w293]
            tunnel: w255 -> [w292]
            tunnel: w265 -> [_]
            shift-right: [w280] -> w263
            shift-left: w261 -> [w288]
            tunnel: w250 -> [w278]
            tunnel: w249 -> [w273]
            stop <- w276 stop-if-true
            w274 = u32 1 items=["Horizontal", "Vertical", "Central", "1st Diagonal", "2nd Diagonal"] ("Type of Symmetry")
            n156 = node-c288() -> (→"ROI循环持续时间":i64)  [unwired: 2 out]
            n157 = event shown="[1] 键按下" {
              selector: _ -> [_ _ _]
              dyn-events: _ -> [_ _ _]
              timeout: 0 -> [_ _ _]
              tunnel: [w313 w314 w453] -> w294
              tunnel: w296 -> [w313 w323 w444]
              tunnel: w288 -> [w312 w316 w443]
              tunnel: [w312 w315 w452] -> w280
              event Timeout {
                n158 = event-data() -> ()  [unwired: 3 out]
              }
              event Key Down {
                n159 = event-data() -> ("VKey"=w324:T20)  [unwired: 10 out]
                n160 = local read "blank of eye"() -> (w318:T4)
                n161 = Unbundle By Name(w318) -> ("NO. of Eyes"=w322:u16, "单选按钮"=w321:enum32{"单选选项1", "单选选项2"})
                n162 = Equal To 0?(x=w322) -> (x = 0?=w320:bool)
                n163 = Equal To 0?(x=w321) -> (x = 0?=w319:bool)
                n164 = Or(x=w320, y=w319) -> (x .or. y?=w317:bool)
                n165 = case shown="\"Left\"" w324 {
                  tunnel: w323 -> [w326 w330 w357 w388 w416]
                  tunnel: w317 -> [_ w327 w356 w389 w415]
                  tunnel: w316 -> [w325 w329 w358 w387 w414]
                  tunnel: [w325 w331 w359 w386 w418] -> w315
                  tunnel: [w326 w328 w360 w385 w417] -> w314
                  frame "ASCII", Default {
                  }
                  frame "Left" {
                    n166 = case shown="假" w327 {
                      tunnel: w330 -> [w336 w348]
                      tunnel: w329 -> [w338 w347]
                      tunnel: [w337 w347] -> w331
                      tunnel: [w336 w349] -> w328
                      frame False {
                        n167 = call "RectangleToCenter.vi"("rectangle"=w336) -> ("hight"=w340:i32, "width"=w343:i32)  [unwired: 9 out]
                        n168 = call "RectangleToCenter.vi"("rectangle"=w338) -> ("hight"=w333:i32, "width"=w334:i32, "center"=w339:cluster{i32, i32})  [unwired: 8 out]
                        n169 = Bundle("width"=w343, "hight"=w340) -> (w341:cluster{"width":i32, "hight":i32})  [unwired: 1 out]
                        n170 = Subtract(x=w334, y=2) -> (x-y=w332:i32)
                        n171 = property on="eye1" class="Pict"("Draw Area Size"=w341) -> ()  [unwired: 2 in, 2 out]
                        n172 = call "CenterToRectangle.vi"("hight"=w333, "width"=w332, "center"=w339) -> ("rectangle"=w337:cluster{i32, i32, i32, i32})  [unwired: 8 out]
                        n173 = Bundle(w332, "hight"=w333) -> (w342:cluster{i32, "hight":i32})  [unwired: 1 out]
                        n174 = property on="eye2" class="Pict"("Draw Area Size"=w342) -> ()  [unwired: 2 in, 2 out]
                      }
                      frame True {
                        n175 = call "RectangleToCenter.vi"("rectangle"=w348) -> ("hight"=w346:i32, "width"=w345:i32, "center"=w355:cluster{i32, i32})  [unwired: 8 out]
                        n176 = call "RectangleToCenter.vi"("rectangle"=w347) -> ("hight"=w353:i32, "width"=w352:i32)  [unwired: 9 out]
                        n177 = Bundle("width"=w352, "hight"=w353) -> (w351:cluster{"width":i32, "hight":i32})  [unwired: 1 out]
                        n178 = Subtract(x=w345, y=2) -> (x-y=w344:i32)
                        n179 = call "CenterToRectangle.vi"("hight"=w346, "width"=w344, "center"=w355) -> ("rectangle"=w349:cluster{i32, i32, i32, i32})  [unwired: 8 out]
                        n180 = Bundle(w344, "hight"=w346) -> (w350:cluster{i32, "hight":i32})  [unwired: 1 out]
                        n181 = property on="eye2" class="Pict"("Draw Area Size"=w351) -> ()  [unwired: 2 in, 2 out]
                        n182 = property on="eye1" class="Pict"("Draw Area Size"=w350) -> ()  [unwired: 2 in, 2 out]
                      }
                    }
                  }
                  frame "Right" {
                    n183 = case shown="真" w356 {
                      tunnel: w357 -> [w365 w377]
                      tunnel: w358 -> [w367 w376]
                      tunnel: [w366 w376] -> w359
                      tunnel: [w365 w378] -> w360
                      frame False {
                        n184 = call "RectangleToCenter.vi"("rectangle"=w365) -> ("hight"=w369:i32, "width"=w372:i32)  [unwired: 9 out]
                        n185 = call "RectangleToCenter.vi"("rectangle"=w367) -> ("hight"=w362:i32, "width"=w363:i32, "center"=w368:cluster{i32, i32})  [unwired: 8 out]
                        n186 = Bundle("width"=w372, "hight"=w369) -> (w370:cluster{"width":i32, "hight":i32})  [unwired: 1 out]
                        n187 = Add(x=w363, y=2) -> (x+y=w361:i32)
                        n188 = property on="eye1" class="Pict"("Draw Area Size"=w370) -> ()  [unwired: 2 in, 2 out]
                        n189 = call "CenterToRectangle.vi"("hight"=w362, "width"=w361, "center"=w368) -> ("rectangle"=w366:cluster{i32, i32, i32, i32})  [unwired: 8 out]
                        n190 = Bundle(w361, "hight"=w362) -> (w371:cluster{i32, "hight":i32})  [unwired: 1 out]
                        n191 = property on="eye2" class="Pict"("Draw Area Size"=w371) -> ()  [unwired: 2 in, 2 out]
                      }
                      frame True {
                        n192 = call "RectangleToCenter.vi"("rectangle"=w377) -> ("hight"=w375:i32, "width"=w374:i32, "center"=w384:cluster{i32, i32})  [unwired: 8 out]
                        n193 = call "RectangleToCenter.vi"("rectangle"=w376) -> ("hight"=w382:i32, "width"=w381:i32)  [unwired: 9 out]
                        n194 = Bundle("width"=w381, "hight"=w382) -> (w380:cluster{"width":i32, "hight":i32})  [unwired: 1 out]
                        n195 = Add(x=w374, y=2) -> (x+y=w373:i32)
                        n196 = call "CenterToRectangle.vi"("hight"=w375, "width"=w373, "center"=w384) -> ("rectangle"=w378:cluster{i32, i32, i32, i32})  [unwired: 8 out]
                        n197 = Bundle(w373, "hight"=w375) -> (w379:cluster{i32, "hight":i32})  [unwired: 1 out]
                        n198 = property on="eye2" class="Pict"("Draw Area Size"=w380) -> ()  [unwired: 2 in, 2 out]
                        n199 = property on="eye1" class="Pict"("Draw Area Size"=w379) -> ()  [unwired: 2 in, 2 out]
                      }
                    }
                  }
                  frame "Up" {
                    n200 = case shown="假" w389 {
                      tunnel: w388 -> [w390 w403]
                      tunnel: w387 -> [w392 w402]
                      tunnel: [w391 w402] -> w386
                      tunnel: [w390 w404] -> w385
                      frame False {
                        n201 = call "RectangleToCenter.vi"("rectangle"=w390) -> ("hight"=w398:i32, "width"=w401:i32)  [unwired: 9 out]
                        n202 = call "RectangleToCenter.vi"("rectangle"=w392) -> ("hight"=w396:i32, "width"=w394:i32, "center"=w395:cluster{i32, i32})  [unwired: 8 out]
                        n203 = Bundle("width"=w401, "hight"=w398) -> (w399:cluster{"width":i32, "hight":i32})  [unwired: 1 out]
                        n204 = Add(x=2 ("y"), y=w396) -> (x+y=w393:i32)
                        n205 = property on="eye1" class="Pict"("Draw Area Size"=w399) -> ()  [unwired: 2 in, 2 out]
                        n206 = call "CenterToRectangle.vi"("hight"=w393, "width"=w394, "center"=w395) -> ("rectangle"=w391:cluster{i32, i32, i32, i32})  [unwired: 8 out]
                        n207 = Bundle("width"=w394, w393) -> (w400:cluster{"width":i32, i32})  [unwired: 1 out]
                        n208 = property on="eye2" class="Pict"("Draw Area Size"=w400) -> ()  [unwired: 2 in, 2 out]
                      }
                      frame True {
                        n209 = call "RectangleToCenter.vi"("rectangle"=w403) -> ("hight"=w409:i32, "width"=w412:i32, "center"=w411:cluster{i32, i32})  [unwired: 8 out]
                        n210 = call "RectangleToCenter.vi"("rectangle"=w402) -> ("hight"=w408:i32, "width"=w407:i32)  [unwired: 9 out]
                        n211 = Bundle("width"=w407, "hight"=w408) -> (w406:cluster{"width":i32, "hight":i32})  [unwired: 1 out]
                        n212 = Add(x=w409, y=2) -> (x+y=w413:i32)
                        n213 = call "CenterToRectangle.vi"("hight"=w413, "width"=w412, "center"=w411) -> ("rectangle"=w404:cluster{i32, i32, i32, i32})  [unwired: 8 out]
                        n214 = Bundle("width"=w412, w413) -> (w405:cluster{"width":i32, i32})  [unwired: 1 out]
                        n215 = property on="eye2" class="Pict"("Draw Area Size"=w406) -> ()  [unwired: 2 in, 2 out]
                        n216 = property on="eye1" class="Pict"("Draw Area Size"=w405) -> ()  [unwired: 2 in, 2 out]
                      }
                    }
                  }
                  frame "Down" {
                    n217 = case shown="假" w415 {
                      tunnel: w416 -> [w421 w432]
                      tunnel: w414 -> [w423 w431]
                      tunnel: [w422 w431] -> w418
                      tunnel: [w421 w433] -> w417
                      frame False {
                        n218 = call "RectangleToCenter.vi"("rectangle"=w421) -> ("hight"=w427:i32, "width"=w430:i32)  [unwired: 9 out]
                        n219 = call "RectangleToCenter.vi"("rectangle"=w423) -> ("hight"=w420:i32, "width"=w425:i32, "center"=w426:cluster{i32, i32})  [unwired: 8 out]
                        n220 = Bundle("width"=w430, "hight"=w427) -> (w428:cluster{"width":i32, "hight":i32})  [unwired: 1 out]
                        n221 = Subtract(x=w420, y=2) -> (x-y=w424:i32)
                        n222 = property on="eye1" class="Pict"("Draw Area Size"=w428) -> ()  [unwired: 2 in, 2 out]
                        n223 = call "CenterToRectangle.vi"("hight"=w424, "width"=w425, "center"=w426) -> ("rectangle"=w422:cluster{i32, i32, i32, i32})  [unwired: 8 out]
                        n224 = Bundle("width"=w425, w424) -> (w429:cluster{"width":i32, i32})  [unwired: 1 out]
                        n225 = property on="eye2" class="Pict"("Draw Area Size"=w429) -> ()  [unwired: 2 in, 2 out]
                      }
                      frame True {
                        n226 = call "RectangleToCenter.vi"("rectangle"=w432) -> ("hight"=w438:i32, "width"=w441:i32, "center"=w440:cluster{i32, i32})  [unwired: 8 out]
                        n227 = call "RectangleToCenter.vi"("rectangle"=w431) -> ("hight"=w437:i32, "width"=w436:i32)  [unwired: 9 out]
                        n228 = Bundle("width"=w436, "hight"=w437) -> (w435:cluster{"width":i32, "hight":i32})  [unwired: 1 out]
                        n229 = Subtract(x=w438, y=2) -> (x-y=w442:i32)
                        n230 = call "CenterToRectangle.vi"("hight"=w442, "width"=w441, "center"=w440) -> ("rectangle"=w433:cluster{i32, i32, i32, i32})  [unwired: 8 out]
                        n231 = Bundle("width"=w441, w442) -> (w434:cluster{"width":i32, i32})  [unwired: 1 out]
                        n232 = property on="eye2" class="Pict"("Draw Area Size"=w435) -> ()  [unwired: 2 in, 2 out]
                        n233 = property on="eye1" class="Pict"("Draw Area Size"=w434) -> ()  [unwired: 2 in, 2 out]
                      }
                    }
                  }
                }
              }
              event "new picture": Mouse Down {
                n234 = event-data() -> ()  [unwired: 2 out]
                n235 = call "RectangleToCenter.vi"("rectangle"=w444) -> ("hight"=w446:i32, "width"=w445:i32)  [unwired: 9 out]
                n236 = call "RectangleToCenter.vi"("rectangle"=w443) -> ("hight"=w450:i32, "width"=w449:i32)  [unwired: 9 out]
                n237 = Bundle("width"=w445, "hight"=w446) -> (w447:cluster{"width":i32, "hight":i32})  [unwired: 1 out]
                n238 = Bundle("width"=w449, "hight"=w450) -> (w448:cluster{"width":i32, "hight":i32})  [unwired: 1 out]
                n239 = property on="eye1" class="Pict"("Draw Area Size"=w447) -> ()  [unwired: 2 in, 2 out]
                n240 = property on="eye2" class="Pict"("Draw Area Size"=w448) -> ()  [unwired: 2 in, 2 out]
                n241 = local read "blank of eye"() -> (w459:T4)
                n242 = Unbundle By Name(w459) -> ("NO. of Eyes"=w458:u16, "单选按钮"=w457:enum32{"单选选项1", "单选选项2"})
                n243 = Equal To 0?(x=w458) -> (x = 0?=w456:bool)
                n244 = Equal To 0?(x=w457) -> (x = 0?=w455:bool)
                n245 = property on="new picture" class="Pict"() -> ("Mouse"=w460:T21)  [unwired: 2 in, 2 out]
                n246 = Unbundle By Name(w460) -> ("Mouse Position"=w451:cluster{"X":i32, "Y":i32})
                n247 = Or(x=w456, y=w455) -> (x .or. y?=w454:bool)
                n248 = case shown="假" w454 {
                  tunnel: [w466 w467] -> w453
                  tunnel: [w461 w472] -> w452
                  tunnel: w444 -> [w466 w471]
                  tunnel: w443 -> [w463 w472]
                  tunnel: w451 -> [w462 w468]
                  frame False {
                    n249 = call "RectangleToCenter.vi"("rectangle"=w463) -> ("hight"=w465:i32, "width"=w464:i32)  [unwired: 9 out]
                    n250 = call "CenterToRectangle.vi"("hight"=w465, "width"=w464, "center"=w462) -> ("rectangle"=w461:cluster{i32, i32, i32, i32})  [unwired: 8 out]
                  }
                  frame True {
                    n251 = call "RectangleToCenter.vi"("rectangle"=w471) -> ("hight"=w470:i32, "width"=w469:i32)  [unwired: 9 out]
                    n252 = call "CenterToRectangle.vi"("hight"=w470, "width"=w469, "center"=w468) -> ("rectangle"=w467:cluster{i32, i32, i32, i32})  [unwired: 8 out]
                  }
                }
              }
            }
            "rectangle2" <- w280
            "rectangle1" <- w294
            n253 = Wait on Notification(notifier=w278) -> (notification=w277:cluster{"Image Pixels (U8)":u8[][], "停止":bool})  [unwired: 1 in, 5 out]
            n254 = Unbundle(w277) -> ("Image Pixels (U8)"=w275:u8[][], "停止"=w276:bool)
            n255 = case shown="真" TRUE {
              tunnel: w275 -> [w300 w306]
              tunnel: [w300 w304] -> w271
              tunnel: w274 -> [_ w302]
              tunnel: w273 -> [_ w301]
              frame False {
              }
              frame True {
                n256 = call "IMAQ ArrayToImage"("Image Pixels (U8)"=w306, "Image"=w301) -> ("Image Out"=w305:T3)  [unwired: 4 in, 5 out]
                n257 = call "IMAQ Symmetry"("Type of Symmetry"=w302, "Image Src"=w305) -> ("Image Dst Out"=w303:T3)  [unwired: 2 in, 2 out]
                n258 = call "IMAQ ImageToArray"("Image"=w303) -> ("Image Pixels (U8)"=w304:u8[][])  [unwired: 2 in, 5 out]
              }
            }
            n259 = call <vilib>:"Flatten Pixmap.vi"("colors"=w298, "8-bit pixmap"=w271) -> ("image data"=w281:T14)  [unwired: 4 in, 5 out]
            n260 = Unbundle By Name("blank of eye") -> ("NO. of Eyes"=w284:u16, "eye1"=w289:u32, "eye2"=w285:u32)
            n261 = call <vilib>:"Draw Flattened Pixmap.vi"("image data"=w281) -> ("new picture"=w295:picture)  [unwired: 1 in, 7 out]
            n262 = Not Equal To 0?(x=w284) -> (x != 0?=w283:bool)
            n263 = call <vilib>:"Get Image Subset.vi"("subset rect"=w280, "image data"=w281) -> ("image subset"=w279:T14)  [unwired: 5 out]
            n264 = call <vilib>:"Get Image Subset.vi"("subset rect"=w294, "image data"=w281) -> ("image subset"=w282:T14)  [unwired: 5 out]
            n265 = call <vilib>:"Draw Rect.vi"("picture"=w295, "rect"=w294, "color(black)"=w289) -> ("new picture"=w287:picture)  [unwired: 2 in, 4 out]
            n266 = case shown="真" w283 {
              tunnel: w287 -> [w307 w311]
              tunnel: [w307 w310] -> w286
              tunnel: w280 -> [_ w309]
              tunnel: w285 -> [_ w308]
              frame False {
              }
              frame True {
                n267 = call <vilib>:"Draw Rect.vi"("picture"=w311, "rect"=w309, "color(black)"=w308) -> ("new picture"=w310:picture)  [unwired: 2 in, 4 out]
              }
            }
            "new picture" <- w286
            n268 = Bundle("image subset"=w282, "image subset"=w279, "停止"=w276) -> (w291:T22)  [unwired: 1 out]
            n269 = Send Notification(notification=w291, notifier=w293, error in (no error)=w292) -> ()  [unwired: 2 out]
            n270 = node-c288() -> ()  [unwired: 2 out]
          }
          n271 = node-c288(w269) -> ()  [unwired: 1 out]
        }
      }
      n272 = flat-sequence {
        frame #0 {
          w573 = T14 {"image type"=0, "image depth"=0, "image"=[], "mask"=[], "colors"=[], "Rectangle"={"left"=0, "top"=0, "right"=0, "bottom"=0}} ("image subset")
          w582 = T13 0 items=["Grayscale (U8)", "Grayscale (I16)", "Grayscale (SGL)", "Complex (CSG)", "RGB (U32)", "HSL (U32)", "RGB (U64)", "Grayscale (U16)"] ("Image Type")
          n273 = local read "CR Threshold 2"() -> (w578:u8)
          n274 = local read "Pupil Threshold 2"() -> (w577:u8)
          n275 = Bundle("image subset"=w573, "image subset"=w573, FALSE) -> (w571:T15)  [unwired: 1 out]
          n276 = call "IMAQ Create"("Image Name"="EYE2", "Image Type"=w582) -> ("New Image"=w581:T3)  [unwired: 2 in, 2 out]
          n277 = call "ThresholdColour.vi"("Pupil Threshold"=w577, "HighLight Spot Threshold"=w578) -> ("colors"=w579:u32[])  [unwired: 9 out]
          n278 = Obtain Notifier(name (unnamed)="eyeData2" ("Image Name"), notification data type=dbl[] [] ("添加的数组")) -> (notifier out=w575:refnum<notifier>, error out=w574:errorcluster)  [unwired: 2 in, 1 out]
          n279 = Obtain Notifier(name (unnamed)="EYE1" ("Image Name"), notification data type=w571) -> (notifier out=w569:refnum<notifier>, error out=w568:errorcluster)  [unwired: 2 in, 1 out]
          n280 = node-c288() -> (w584:T5)  [unwired: 4 out]
          n281 = timed-loop {
            timing: w584 -> [_]
            timing-out: [_] -> w583
            shift-right: [w601] -> _
            shift-left: w579 -> [w600]
            tunnel: w581 -> [w597]
            tunnel: w569 -> [w595]
            tunnel: w568 -> [w594]
            tunnel: w575 -> [w591]
            tunnel: w574 -> [w590]
            shift-right: [w586] -> _
            shift-left: T8 {"pupil-CR array output"={[], []}, "CR array output"={[], []}, "pupil array output 3"={[], []}} ("data array output") -> [w585]
            stop <- w593 stop-if-true
            n282 = node-c288() -> (→"数据处理循环持续时间 2":i64)  [unwired: 1 out]
            n283 = Wait on Notification(notifier=w595, error in (no error)=w594) -> (notification=w596:T15)  [unwired: 5 out]
            n284 = local read "blank of eye"() -> (w589:T4)
            n285 = Unbundle(w596) -> ("image subset"=w592:T14, w593:bool)  [unwired: 1 out]
            n286 = Unbundle By Name(w589) -> ("NO. of Eyes"=w588:u16)
            n287 = Not Equal To 0?(x=w588) -> (x != 0?=w587:bool)
            n288 = event shown="[1] \"CR Threshold 2\", \"Pupil Threshold 2\": 值改变" {
              selector: _ -> [_ _]
              dyn-events: _ -> [_ _]
              timeout: 0 -> [_ _]
              tunnel: "CR Threshold 2" -> [_ w641]
              tunnel: "Pupil Threshold 2" -> [_ w640]
              tunnel: [w638 w639] -> w601
              tunnel: w600 -> [w638 _]
              event Timeout {
                n289 = event-data() -> ()  [unwired: 3 out]
              }
              event "CR Threshold 2", "Pupil Threshold 2": Value Change {
                n290 = event-data() -> ()  [unwired: 7 out]
                n291 = call "ThresholdColour.vi"("Pupil Threshold"=w640, "HighLight Spot Threshold"=w641) -> ("colors"=w639:u32[])  [unwired: 9 out]
              }
            }
            n292 = case shown="真" w587 {
              tunnel: w600 -> [_ w637]
              tunnel: "CR Threshold 2" -> [_ w629]
              tunnel: "Pupil Threshold 2" -> [_ w628]
              tunnel: w597 -> [_ w624]
              tunnel: w592 -> [_ w623]
              tunnel: w591 -> [w607 w622]
              tunnel: w590 -> [w606 w621]
              tunnel: [w605 w620] -> w586
              tunnel: w585 -> [w605 w619]
              frame False {
                n293 = Send Notification(notification=dbl[] [0.0, 0.0, 0.0, 0.0, 0.0, 0.0] ("通知"), notifier=w607, error in (no error)=w606) -> ()  [unwired: 2 out]
              }
              frame True {
                w631 = 5 ("pixel")
                n294 = call <vilib>:"Unflatten Pixmap.vi"("image data"=w623) -> ("8-bit pixmap"=w634:u8[][])  [unwired: 10 out]
                n295 = local read "rectangle2"() -> (w615:T2)
                n296 = call "rectangleCheck0.vi"("rectangle"=w615) -> ("rectangle out"=w614:cluster{"x1":i32, "y1":i32})  [unwired: 10 out]
                n297 = call "IMAQ ArrayToImage"("Image Pixels (U8)"=w634, "Image"=w624) -> ("Image Out"=w633:T3)  [unwired: 4 in, 5 out]
                n298 = call "Pupil&CR_Detecter.vi"("Image Name"="ellipse-eye2", "Pupil Threshold"=w628, "HighLight Spot Threshold"=w629, "image input"=w633) -> ("valid fit"=→"valid fit 2":T16, "Image Dst Out"=w627:T3, "pupil Circles Data"=w612:cluster{"Pos. X":sgl, "Pos. Y":sgl}, "CR Circles Data"=w613:cluster{"Pos. X":sgl, "Pos. Y":sgl}, "Image Out"=→"Image 2":T3)  [unwired: 3 out]
                n299 = Add(x=w614, y=w613) -> (x+y=w609:cluster{sgl, sgl})
                n300 = Add(x=w614, y=w612) -> (x+y=w608:cluster{sgl, sgl})
                n301 = Bundle("CR Circles Data"=w613, "pupil Circles Data"=w612) -> ()  [unwired: 2 out]
                n302 = call "IMAQ ImageToArray"("Image"=w627) -> ("Image Pixels (U8)"=w626:u8[][])  [unwired: 2 in, 5 out]
                n303 = call <vilib>:"Flatten Pixmap.vi"("colors"=w637, "8-bit pixmap"=w626) -> ("image data"=w636:T14)  [unwired: 4 in, 5 out]
                n304 = call "EyePositionBin.vi"("gaze Threshold"="gaze Threshold 2", "pupil input"=w608, "CR input"=w609, "data array input"=w619) -> ("data array output"=w620:T8, "gaze"=→"gazing 2":bool, "eyeposition array"=w610:dbl[])  [unwired: 1 in, 4 out]
                n305 = Send Notification(notification=w610, notifier=w622, error in (no error)=w621) -> ()  [unwired: 2 out]
                n306 = call <vilib>:"Draw Flattened Pixmap.vi"("image data"=w636) -> ("new picture"=w635:picture)  [unwired: 1 in, 7 out]
                n307 = call "DrawCross.vi"("pixel"=w631, "position"=w613, "picture input"=w635) -> ("picture Output"=w632:picture)  [unwired: 1 in, 7 out]
                n308 = call "DrawCross.vi"("pixel"=w631, "position"=w612, "picture input"=w632) -> ("picture Output"=→"eye2":picture)  [unwired: 1 in, 7 out]
              }
            }
            n309 = node-c288() -> ()  [unwired: 2 out]
          }
          n310 = node-c288(w583) -> ()  [unwired: 1 out]
        }
      }
      n311 = call "IMAQ Create"("Image Name"="symmetry", "Image Type"=w164) -> ("New Image"=w166:T3)  [unwired: 2 in, 2 out]
    }
    frame #2 {
      n312 = flat-sequence {
        tunnel: w652 -> [w655]
        frame #0 {
          n313 = dll-call lib="PTH1]abs CDocuments and Settingspan桌面workeye tracker\nHikvision Dll\nDs40xxSDK.dll" fn="DeInitDSPs"(path in=w655) -> ("返回类型"=→"返回类型":i32)  [unwired: 2 in, 2 out]
        }
      }
      n314 = flat-sequence {
        tunnel: w654 -> [w730]
        tunnel: w653 -> [w702]
        frame #0 {
          w657 = "CheckEyes" ("section")
          w677 = "Threshold" ("section")
          w693 = "VideoCardPara" ("section")
          w713 = "Eye2Rectangle" ("section")
          w718 = "Eye1Rectangle" ("section")
          n315 = Unbundle(w702) -> ("value"=w701:i32, "value"=w700:i32, "value"=w699:i32, "value"=w698:i32)
          n316 = local read "Pupil Threshold1"() -> (w683:u8)
          n317 = local read "CR Threshold1"() -> (w684:u8)
          n318 = Current VI's Path() -> (path=w736:path)
          n319 = Strip Path(path=w736) -> (stripped path=w735:path)  [unwired: 1 out]
          n320 = local read "blank of eye"() -> (w674:T4)
          n321 = Build Path(base path=w735, name or relative path="parameter.ini" ("名称或相对路径")) -> (appended path=w733:path)
          n322 = call <vilib>:"Open Config Data (compatibility).vi"("configuration file path"=w733) -> ("refnum"=w732:T9)  [unwired: 8 in, 2 out]
          n323 = Unbundle(w730) -> ("value"=w727:i32, "value"=w725:i32, "value"=w722:i32, "value"=w719:i32)
          n324 = Unbundle By Name(w674) -> ("NO. of Eyes"=w663:u16, "单选按钮"=w662:enum32{"单选选项1", "单选选项2"}, "eye1"=w661:u32, "eye2"=w660:u32)
          n325 = call-poly <vilib>:"Write Key.vi"("section"=w718, "value"=w727, "key"="x1", "refnum"=w732) -> ("error out"=w729:errorcluster, "refnum out"=w728:T9)  [unwired: 1 in, 5 out]
          n326 = call-poly <vilib>:"Write Key.vi"("section"=w718, "error in (no error)"=w729, "value"=w725, "key"="y1", "refnum"=w728) -> ("error out"=w724:errorcluster, "refnum out"=w723:T9)  [unwired: 5 out]
          n327 = local read "VideoPara"() -> (w690:cluster{"Brightness":i32, "Contrast":i32})
          n328 = call-poly <vilib>:"Write Key.vi"("section"=w718, "error in (no error)"=w724, "value"=w722, "key"="x2", "refnum"=w723) -> ("error out"=w721:errorcluster, "refnum out"=w720:T9)  [unwired: 5 out]
          n329 = Unbundle By Name(w690) -> ("Brightness"=w689:i32, "Contrast"=w688:i32)
          n330 = local read "Pupil Threshold 2"() -> (w676:u8)
          n331 = local read "CR Threshold 2"() -> (w681:u8)
          n332 = call-poly <vilib>:"Write Key.vi"("section"=w718, "error in (no error)"=w721, "value"=w719, "key"="y2", "refnum"=w720) -> ("error out"=w703:errorcluster, "refnum out"=w704:T9)  [unwired: 5 out]
          n333 = call-poly <vilib>:"Write Key.vi"("section"=w713, "error in (no error)"=w703, "value"=w701, "key"="x1", "refnum"=w704) -> ("error out"=w706:errorcluster, "refnum out"=w707:T9)  [unwired: 5 out]
          n334 = call-poly <vilib>:"Write Key.vi"("section"=w713, "error in (no error)"=w706, "value"=w700, "key"="y1", "refnum"=w707) -> ("error out"=w709:errorcluster, "refnum out"=w710:T9)  [unwired: 5 out]
          n335 = call-poly <vilib>:"Write Key.vi"("section"=w713, "error in (no error)"=w709, "value"=w699, "key"="x2", "refnum"=w710) -> ("error out"=w711:errorcluster, "refnum out"=w712:T9)  [unwired: 5 out]
          n336 = call-poly <vilib>:"Write Key.vi"("section"=w713, "error in (no error)"=w711, "value"=w698, "key"="y2", "refnum"=w712) -> ("error out"=w696:errorcluster, "refnum out"=w697:T9)  [unwired: 5 out]
          n337 = call-poly <vilib>:"Write Key.vi"("section"=w693, "error in (no error)"=w696, "value"=w689, "key"="Brightness", "refnum"=w697) -> ("error out"=w694:errorcluster, "refnum out"=w695:T9)  [unwired: 5 out]
          n338 = call-poly <vilib>:"Write Key.vi"("section"=w693, "error in (no error)"=w694, "value"=w688, "key"="Contrast", "refnum"=w695) -> ("refnum out"=w675:T9)  [unwired: 6 out]
          n339 = call-poly <vilib>:"Write Key.vi"("section"=w677, "value"=w684, "key"="eye1CR", "refnum"=w675) -> ("refnum out"=w686:T9)  [unwired: 1 in, 6 out]
          n340 = call-poly <vilib>:"Write Key.vi"("section"=w677, "value"=w683, "key"="eye1pupil", "refnum"=w686) -> ("refnum out"=w680:T9)  [unwired: 1 in, 6 out]
          n341 = call-poly <vilib>:"Write Key.vi"("section"=w677, "value"=w681, "key"="eye2CR", "refnum"=w680) -> ("refnum out"=w679:T9)  [unwired: 1 in, 6 out]
          n342 = call-poly <vilib>:"Write Key.vi"("section"=w677, "value"=w676, "key"="eye2pupil", "refnum"=w679) -> ("refnum out"=w659:T9)  [unwired: 1 in, 6 out]
          n343 = call-poly <vilib>:"Write Key.vi"("section"=w657, "value"=w663, "key"="NO.of eyes", "refnum"=w659) -> ("error out"=w672:errorcluster, "refnum out"=w671:T9)  [unwired: 1 in, 5 out]
          n344 = call-poly <vilib>:"Write Key.vi"("section"=w657, "error in (no error)"=w672, "value"=w662, "key"="单选按钮", "refnum"=w671) -> ("error out"=w670:errorcluster, "refnum out"=w669:T9)  [unwired: 5 out]
          n345 = call-poly <vilib>:"Write Key.vi"("section"=w657, "error in (no error)"=w670, "value"=w661, "key"="eye1", "refnum"=w669) -> ("error out"=w668:errorcluster, "refnum out"=w667:T9)  [unwired: 5 out]
          n346 = call-poly <vilib>:"Write Key.vi"("section"=w657, "error in (no error)"=w668, "value"=w660, "key"="eye2", "refnum"=w667) -> ("refnum out"=w658:T9)  [unwired: 6 out]
          n347 = call <vilib>:"Close Config Data.vi"("error in (no error)"=w696, "refnum"=w658) -> ()  [unwired: 1 in, 9 out]
        }
      }
      n348 = Current VI's Path() -> (path=w649:path)
      n349 = Strip Path(path=w649) -> (stripped path=w650:path)  [unwired: 1 out]
      n350 = global read "全局 1.vi" "9dots"() -> (w647:dbl[][])
      n351 = Build Path(base path=w650, name or relative path="9dots.ini" ("名称或相对路径")) -> (appended path=w648:path)
      n352 = call-poly <vilib>:"Write To Spreadsheet File.vi"("2D data"=w647, "file path (dialog if empty)"=w648) -> ()  [unwired: 4 in, 3 out]
    }
  }
